vi "RT Loop - Acquisition and Logging.vi"(8 "error in (no error)":errorcluster, 9 "Acquisition and Logging Configuration":T1={"Data Rate"=1, "Samples per Read"=0, "Number of Reads to Save"=0, "Data File Name"="", "TDMS Properties"=[], "Number of Channels"=4, "Channel Scale Array"=[0.0, 0.0, 0.0, 0.0, 1.0, 1.0, 1.0, 1.0], "Channel Names"=[], "Trigger - RMS Value"=0.0, "Trigger - Channel"=0, "Trigger - Time (Minute)"=0} {"Data Rate" items=["51.200 kS/s (NI 9234)"=1, "25.600 kS/s (NI 9234)"=2, "17.067 kS/s (NI 9234)"=3, "12.800 kS/s (NI 9234)"=4, "10.240 kS/s (NI 9234)"=5, "8.533 kS/s (NI 9234)"=6, "7.314 kS/s (NI 9234)"=7, "6.400 kS/s (NI 9234)"=8, "5.689 kS/s (NI 9234)"=9, "5.120 kS/s (NI 9234)"=10, "4.654 kS/s (NI 9234)"=11, "4.267 kS/s (NI 9234)"=12, "3.938 kS/s (NI 9234)"=13, "3.657 kS/s (NI 9234)"=14, "3.413 kS/s (NI 9234)"=15, "3.200 kS/s (NI 9234)"=16, "3.012 kS/s (NI 9234)"=17, "2.845 kS/s (NI 9234)"=18, "2.695 kS/s (NI 9234)"=19, "2.560 kS/s (NI 9234)"=20, "2.438 kS/s (NI 9234)"=21, "2.328 kS/s (NI 9234)"=22, "2.226 kS/s (NI 9234)"=23, "2.133 kS/s (NI 9234)"=24, "2.048 kS/s (NI 9234)"=25, "1.969 kS/s (NI 9234)"=26, "1.896 kS/s (NI 9234)"=27, "1.829 kS/s (NI 9234)"=28, "1.765 kS/s (NI 9234)"=29, "1.707 kS/s (NI 9234)"=30, "1.652 kS/s (NI 9234)"=31]}, 10 "Acquisition and Logging Queue":refnum<queue>, 11 "Message Queue":refnum<queue>) -> ()   [LabVIEW 2015]
uses:
  controls/FPGA VI Reference.ctl
  support/Message Queue/Message Queue.lvlib
  Globals/Global - Configuration Options.vi
  Globals/Global - Monitoring Variables.vi
  support/Message Queue/Message Cluster.ctl
  controls/Acquisition and Logging Configuration.ctl
  <vilib>/LabVIEW Targets/FPGA/cRIO/shared/nicrio_ModuleControls/nicrio_cRIO-9234_DataRatesRing2.ctl
  controls/TDMS Properties.ctl
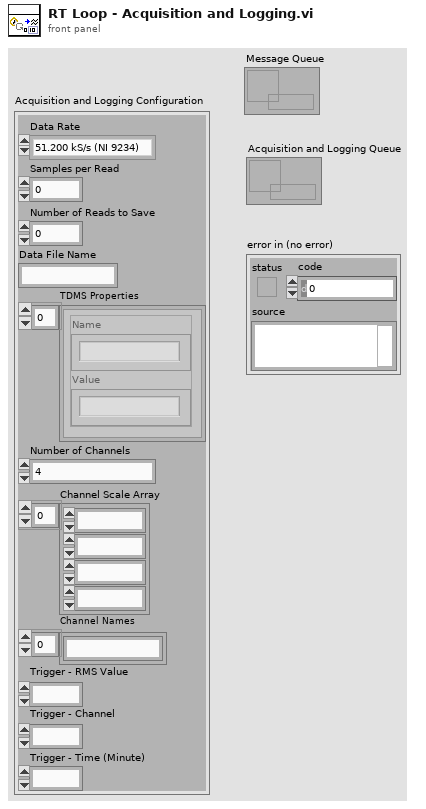
[diagram p1: front panel]
types:
  T1 = typedef "Acquisition and Logging Configuration.ctl" = cluster{"Data Rate":T2, "Samples per Read":i32, "Number of Reads to Save":i32, "Data File Name":string, "TDMS Properties":T3[], "Number of Channels":i32, "Channel Scale Array":fxp<+,24,12>[], "Channel Names":string[], "Trigger - RMS Value":dbl, "Trigger - Channel":i32, "Trigger - Time (Minute)":i32}
  T2 = typedef "nicrio_cRIO-9234_DataRatesRing2.ctl" = u8
  T3 = typedef "TDMS Properties.ctl" = cluster{"Name":string, "Value":string}
  T4 = typedef "FPGA VI Reference.ctl" = refnum<k20>
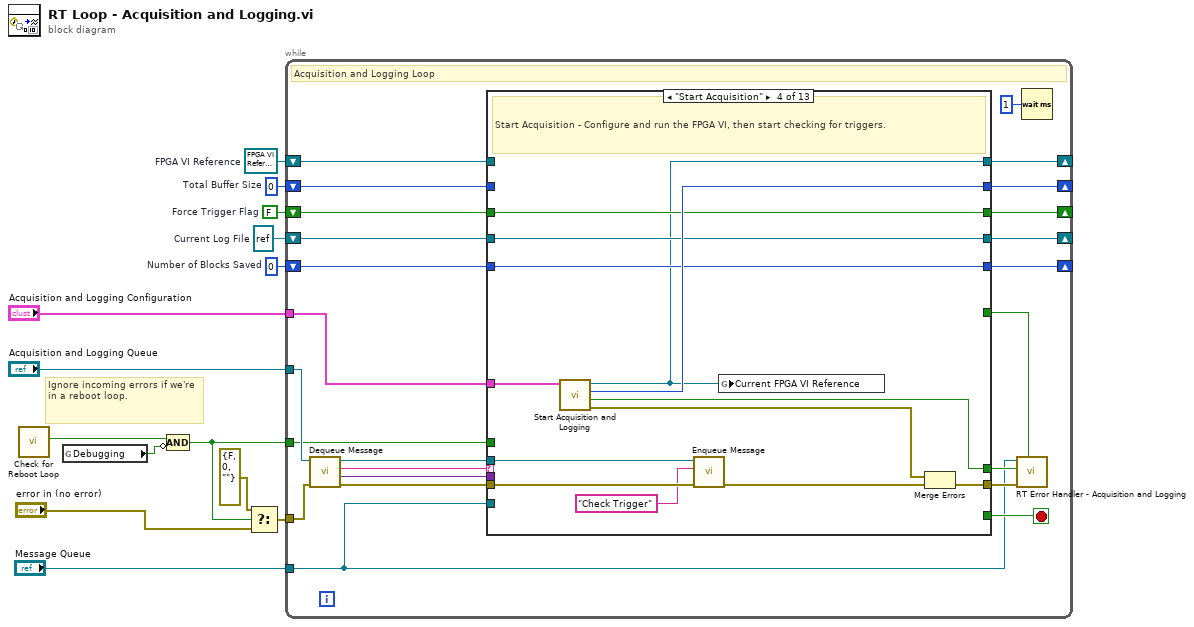
[diagram p0: block diagram]
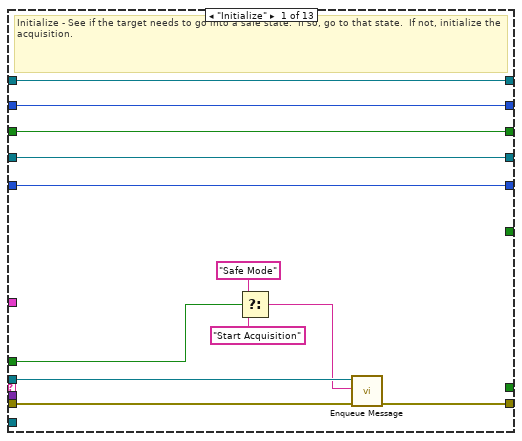
[diagram p2: hidden frame]
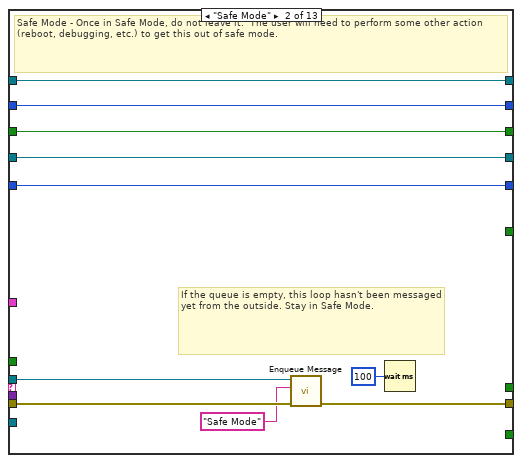
[diagram p3: hidden frame]
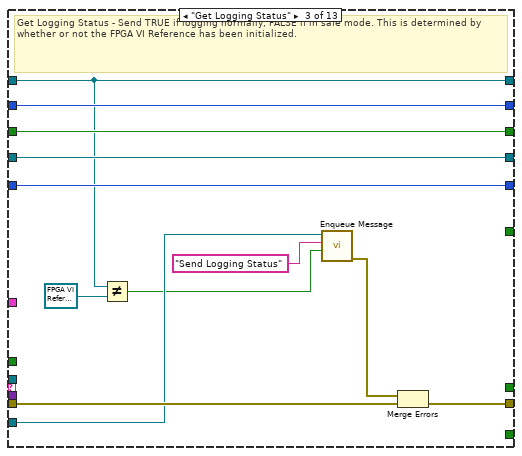
[diagram p4: hidden frame]
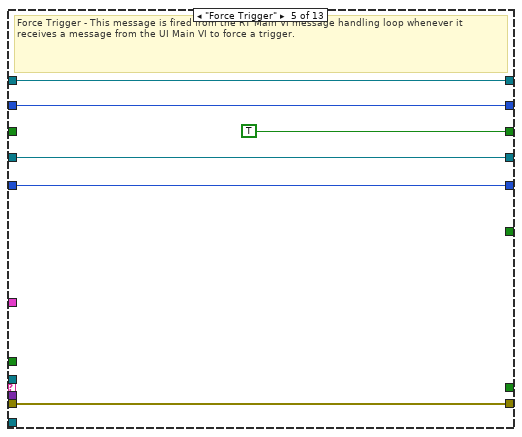
[diagram p5: hidden frame]
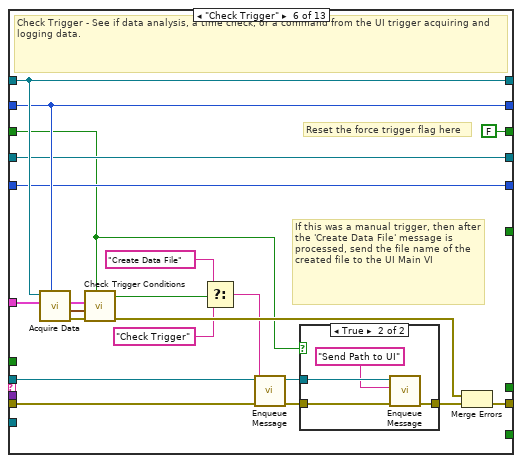
[diagram p6: hidden frame]
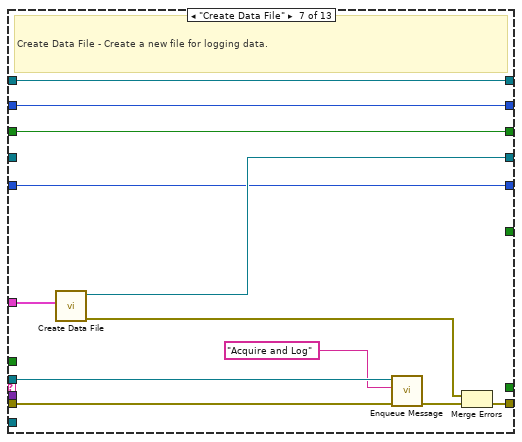
[diagram p8: hidden frame]
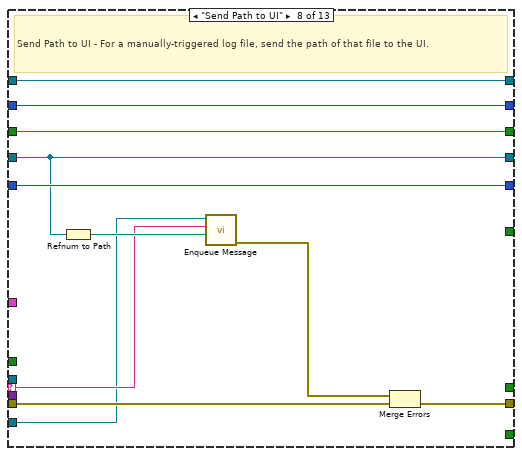
[diagram p9: hidden frame]
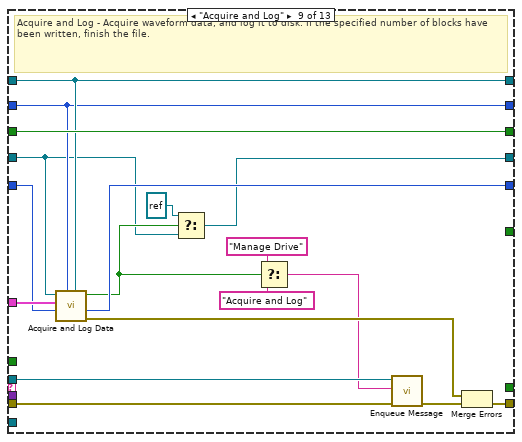
[diagram p10: hidden frame]
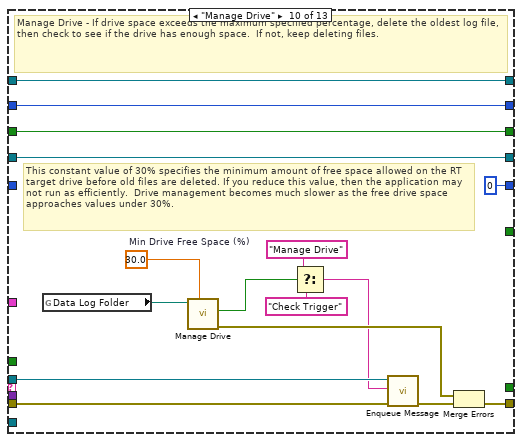
[diagram p11: hidden frame]
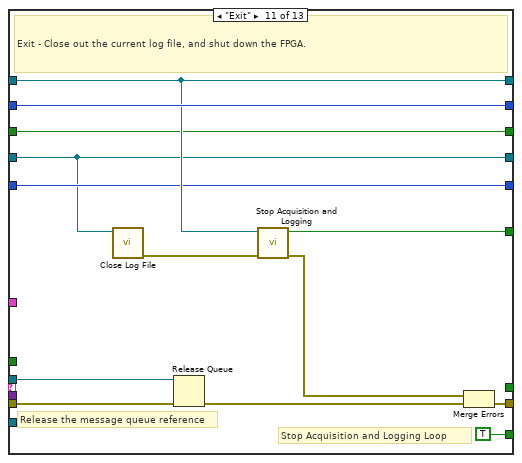
[diagram p12: hidden frame]
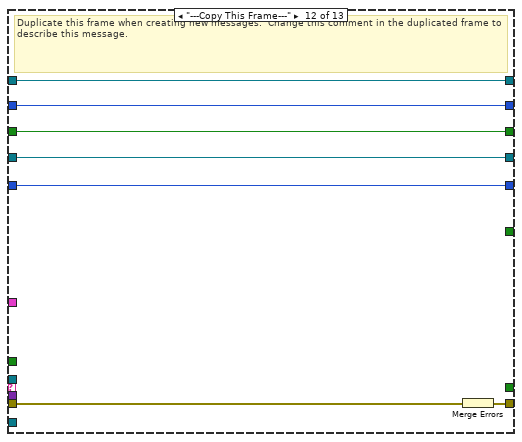
[diagram p13: hidden frame]
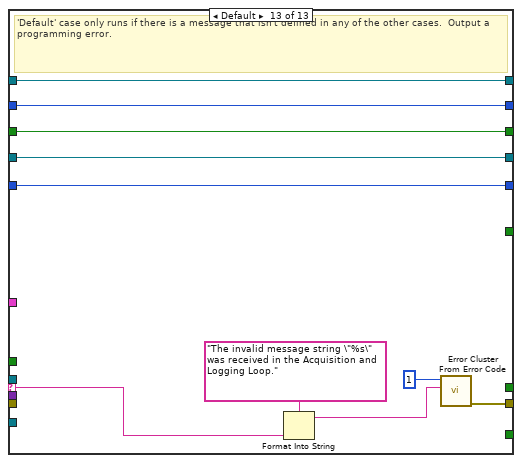
[diagram p14: hidden frame]
diagram:
  w7 = 0  # Number of Blocks Saved
  w8 = refnum<k34> refnum  # Current Log File
  w9 = FALSE  # Force Trigger Flag
  w11 = 0  # Total Buffer Size
  w12 = T4 refnum  # FPGA VI Reference
  # "Ignore incoming errors if we're in a reboot loop."
  n1 = call "Check for Reboot Loop.vi"() -> ("Start in Safe Mode?"=w3:bool)  [unwired: 10 in, 1 out]
  n2 = global read "Global - Configuration Options.vi" "Debugging"() -> (w2:bool)
  n3 = Compound Arithmetic op=AND(w3, invert w2) -> (w1:bool)
  n4 = Select(t=errorcluster {"status"=FALSE, "code"=0, "source"=""}, s=w1, f="error in (no error)") -> (s? t:f=w5:errorcluster)
  n5 = while {
    tunnel: "Acquisition and Logging Queue" -> [w34]
    tunnel: "Message Queue" -> [w18]
    shift-right: [w29] -> _
    shift-left: w12 -> [w31]
    shift-right: [w28] -> _
    shift-left: w11 -> [w30]
    tunnel: "Acquisition and Logging Configuration" -> [w27]
    shift-right: [w23] -> _
    shift-left: w9 -> [w24]
    shift-right: [w21] -> _
    shift-left: w8 -> [w22]
    shift-right: [w19] -> _
    shift-left: w7 -> [w20]
    tunnel: w5 -> [w16]
    tunnel: w1 -> [w15]
    stop <- w38 stop-if-true
    # "Acquisition and Logging Loop"
    n6 = call "Dequeue Message.vi"("error in (no error)"=w16, "Message Queue"=w34) -> ("error out"=w37:errorcluster, "Message Data"=w35:variant, "Message"=w36:string, "dup Message Queue"=w32:refnum<queue>)  [unwired: 6 in]
    n7 = case "Message Cases" shown="\"Start Acquisition\"" w36 {
      selector: w36 -> [_ _ _ _ _ _ _ w133 _ _ _ _ w203]
      tunnel: w32 -> [w47 w57 _ w78 _ w103 w124 _ w155 w167 w187 _ _]
      tunnel: w37 -> [w48 w58 w72 w85 w91 w111 w128 w140 w158 w174 w183 w194 _]
      tunnel: [w40 w56 w64 w83 w91 w110 w127 w131 w157 w170 w184 w193 w201] -> w33
      tunnel: [_ _ _ _ _ _ _ _ _ _ TRUE _ _] -> w38
      tunnel: w35 -> [_ _ _ _ _ _ _ _ _ _ _ _ _]
      tunnel: w31 -> [w50 w60 w67 _ w90 w112 w129 w139 w148 w173 w181 w192 w199]
      tunnel: w30 -> [w49 w59 w71 _ w89 w108 w126 w138 w147 w172 w182 w191 w198]
      tunnel: [w50 w60 w67 w73 w90 w112 w129 w139 w148 w173 w181 w192 w199] -> w29
      tunnel: [w49 w59 w71 w80 w89 w108 w126 w138 w147 w172 w182 w191 w198] -> w28
      tunnel: w27 -> [_ _ _ w84 _ w109 w121 _ w153 _ _ _ _]
      tunnel: [_ _ _ w81 _ _ _ _ _ _ _ _ _] -> w25
      tunnel: w24 -> [w43 w55 w70 w76 _ w92 w122 w137 w154 w160 w179 w190 w197]
      tunnel: [w43 w55 w70 w76 TRUE ("Force Trigger Flag") FALSE ("Force Trigger Flag") w122 w137 w154 w160 w179 w190 w197] -> w23
      tunnel: w22 -> [w42 w54 w69 w75 w88 w98 _ w135 w143 w171 w176 w189 w196]
      tunnel: [w42 w54 w69 w75 w88 w98 w119 w135 w142 w171 w176 w189 w196] -> w21
      tunnel: w20 -> [w41 w53 w68 w74 w86 w97 w118 w136 w146 _ w178 w188 w195]
      tunnel: [w41 w53 w68 w74 w86 w97 w118 w136 w145 0 ("Number of Blocks Saved") w178 w188 w195] -> w19
      tunnel: w18 -> [_ _ w65 _ _ _ _ w132 _ _ _ _ _]
      tunnel: [_ _ _ _ _ _ _ _ _ _ w175 _ _] -> w17
      tunnel: w15 -> [w39 _ _ _ _ _ _ _ _ _ _ _ _]
      frame "Initialize" {
        # "Initialize - See if the target needs to go into a safe state.  If so, go to that state.  If not, initialize the acquisition."
        n8 = Select(t="Safe Mode", s=w39, f="Start Acquisition") -> (s? t:f=w44:string)
        n9 = call "Enqueue Message.vi"("error in (no error)"=w48, "Message"=w44, "Message Queue"=w47) -> ("error out"=w40:errorcluster)  [unwired: 7 in, 1 out]
      }
      frame "Safe Mode" {
        # "If the queue is empty, this loop hasn't been messaged yet from the outside. Stay in Safe Mode."
        # "Safe Mode - Once in Safe Mode, do not leave it.  The user will need to perform some other action (reboot, debugging, etc.) to get this out of safe mode."
        n10 = call "Enqueue Message.vi"("error in (no error)"=w58, "Message"="Safe Mode", "Message Queue"=w57) -> ("error out"=w56:errorcluster)  [unwired: 7 in, 1 out]
        n11 = Wait (ms)(milliseconds to wait=u32 100) -> ()  [unwired: 1 out]
      }
      frame "Get Logging Status" {
        # "Get Logging Status - Send TRUE if logging normally, FALSE if in safe mode. This is determined by whether or not the FPGA VI Reference has been initialized."
        n12 = Not Equal?(x=w67, y=T4 refnum ("FPGA VI Reference")) -> (x != y?=w62:bool)
        n13 = call "Enqueue Message.vi"("Message Data"=w62, "Message"="Send Logging Status", "Message Queue"=w65) -> ("error out"=w63:errorcluster)  [unwired: 7 in, 1 out]
        n14 = Merge Errors(w63, w72) -> (w64:errorcluster)
      }
      frame "Start Acquisition" {
        # "Start Acquisition - Configure and run the FPGA VI, then start checking for triggers."
        n15 = call "Start Acquisition and Logging.vi"("Acquisition and Logging Configuration"=w84) -> ("error out"=w82:errorcluster, "Wait on IRQ Timeout?"=w81:bool, "Total Buffer Size"=w80:i32, "FPGA VI Reference Out"=w73:T4)  [unwired: 7 in]
        n16 = call "Enqueue Message.vi"("error in (no error)"=w85, "Message"="Check Trigger", "Message Queue"=w78) -> ("error out"=w79:errorcluster)  [unwired: 7 in, 1 out]
        n17 = global write "Global - Monitoring Variables.vi" "Current FPGA VI Reference"(w73) -> ()
        n18 = Merge Errors(w82, w79) -> (w83:errorcluster)
      }
      frame "Force Trigger" {
        # "Force Trigger - This message is fired from the RT Main VI message handling loop whenever it receives a message from the UI Main VI to force a trigger."
      }
      frame "Check Trigger" {
        # "If this was a manual trigger, then after the 'Create Data File' message is processed, send the file name of the created file to the UI Main VI"
        # "Reset the force trigger flag here"
        # "Check Trigger - See if data analysis, a time check, or a command from the UI trigger acquiring and logging data."
        n19 = call "Acquire Data.vi"("Total Buffer Size"=w108, "Acquisition and Logging Configuration"=w109, "FPGA VI Reference"=w112) -> ("error out"=w106:errorcluster, "Waveform Data"=w105:waveform(sgl)[], "dup Acquisition and Logging Configuration"=w104:T1)  [unwired: 6 in]
        n20 = call "Check Trigger Conditions.vi"("Force Trigger?"=w92, "error in (no error)"=w106, "Waveform Data"=w105, "Acquisition and Logging Configuration"=w104) -> ("error out"=w107:errorcluster, "Trigger Condition Met?"=w102:bool)  [unwired: 6 in]
        n21 = Select(t="Create Data File", s=w102, f="Check Trigger") -> (s? t:f=w99:string)
        n22 = call "Enqueue Message.vi"("error in (no error)"=w111, "Message"=w99, "Message Queue"=w103) -> ("error out"=w95:errorcluster, "dup Message Queue"=w93:refnum<queue>)  [unwired: 7 in]
        n23 = case shown="True" w92 {
          tunnel: w95 -> [w113 w116]
          tunnel: [w113 w117] -> w94
          tunnel: w93 -> [_ w115]
          frame False {
          }
          frame True {
            n24 = call "Enqueue Message.vi"("error in (no error)"=w116, "Message"="Send Path to UI", "Message Queue"=w115) -> ("error out"=w117:errorcluster)  [unwired: 7 in, 1 out]
          }
        }
        n25 = Merge Errors(w107, w94) -> (w110:errorcluster)
      }
      frame "Create Data File" {
        # "Create Data File - Create a new file for logging data."
        n26 = call "Create Data File.vi"("Acquisition and Logging Configuration"=w121) -> ("error out"=w120:errorcluster, "TDMS File Reference"=w119:refnum<k34>)  [unwired: 9 in]
        n27 = call "Enqueue Message.vi"("error in (no error)"=w128, "Message"="Acquire and Log", "Message Queue"=w124) -> ("error out"=w125:errorcluster)  [unwired: 7 in, 1 out]
        n28 = Merge Errors(w120, w125) -> (w127:errorcluster)
      }
      frame "Send Path to UI" {
        # "Send Path to UI - For a manually-triggered log file, send the path of that file to the UI."
        n29 = Refnum to Path(1:w135) -> (0:w134:path)
        n30 = call "Enqueue Message.vi"("Message Data"=w134, "Message"=w133, "Message Queue"=w132) -> ("error out"=w130:errorcluster)  [unwired: 7 in, 1 out]
        n31 = Merge Errors(w130, w140) -> (w131:errorcluster)
      }
      frame "Acquire and Log" {
        # "Acquire and Log - Acquire waveform data, and log it to disk. If the specified number of blocks have been written, finish the file."
        n32 = call "Acquire and Log Data.vi"("FPGA VI Reference"=w148, "Total Buffer Size"=w147, "Number of Blocks Saved in"=w146, "Acquisition and Logging Configuration"=w153, "TDMS File Reference"=w143) -> ("error out"=w152:errorcluster, "Number of Blocks Saved out"=w145:i32, "Logging Complete?"=w144:bool)  [unwired: 4 in]
        n33 = Select(t=refnum<k34> refnum, s=w144, f=w143) -> (s? t:f=w142:refnum<k34>)
        n34 = Select(t="Manage Drive", s=w144, f="Acquire and Log") -> (s? t:f=w149:string)
        n35 = call "Enqueue Message.vi"("error in (no error)"=w158, "Message"=w149, "Message Queue"=w155) -> ("error out"=w156:errorcluster)  [unwired: 7 in, 1 out]
        n36 = Merge Errors(w152, w156) -> (w157:errorcluster)
      }
      frame "Manage Drive" {
        w169 = 30.0  # Min Drive Free Space (%)
        # "This constant value of 30% specifies the minimum amount of free space allowed on the RT target drive before old files are deleted. If you reduce this value, then the application may not run as efficiently.  Drive management becomes much slower as the free drive space approaches values under 30%."
        # "Manage Drive - If drive space exceeds the maximum specified percentage, delete the oldest log file, then check to see if the drive has enough space.  If not, keep deleting files."
        n37 = global read "Global - Configuration Options.vi" "Data Log Folder"() -> (w159:path)
        n38 = call "Manage Drive.vi"("Min Drive Free Space (%)"=w169, "Data Folder"=w159) -> ("error out"=w166:errorcluster, "Drive Space Below Limit"=w165:bool)  [unwired: 8 in]
        n39 = Select(t="Manage Drive", s=w165, f="Check Trigger") -> (s? t:f=w162:string)
        n40 = call "Enqueue Message.vi"("error in (no error)"=w174, "Message"=w162, "Message Queue"=w167) -> ("error out"=w168:errorcluster)  [unwired: 7 in, 1 out]
        n41 = Merge Errors(w166, w168) -> (w170:errorcluster)
      }
      frame "Exit" {
        # "Stop Acquisition and Logging Loop"
        # "Release the message queue reference"
        # "Exit - Close out the current log file, and shut down the FPGA."
        n42 = call "Close Log File.vi"("Log File"=w176) -> ("error out"=w177:errorcluster)  [unwired: 10 in]
        n43 = Release Queue(queue=w187, error in (no error)=w183) -> (error out=w185:errorcluster)  [unwired: 1 in, 2 out]
        n44 = call "Stop Acquisition and Logging.vi"("error in (no error)"=w177, "FPGA VI Reference"=w181) -> ("error out"=w180:errorcluster, "Stop FPGA Timeout?"=w175:bool)  [unwired: 8 in]
        n45 = Merge Errors(w180, w185) -> (w184:errorcluster)
      }
      frame "---Copy This Frame---" {
        # "Duplicate this frame when creating new messages.  Change this comment in the duplicated frame to describe this message."
        n46 = Merge Errors(w194) -> (w193:errorcluster)
      }
      frame Default {
        # "'Default' case only runs if there is a message that isn't defined in any of the other cases.  Output a programming error."
        n47 = Format Into String(format string="The invalid message string \"%s\" was received in the Acquisition and Logging Loop." ("Unknown Message Error Text"), w203) -> (resulting string=w200:string)  [unwired: 2 in, 1 out]
        n48 = call <vilib>:"Error Cluster From Error Code.vi"("error message (\"\")"=w200, "error code (0)"=1) -> ("error out"=w201:errorcluster)  [unwired: 7 in]
      }
    }
    n49 = call "RT Error Handler - Acquisition and Logging.vi"("Stop FPGA Timeout"=w17, "error in (no error)"=w33, "IRQ Timeout"=w25, "Message Queue"=w18) -> ()  [unwired: 7 in, 1 out]
    n50 = Wait (ms)(milliseconds to wait=u32 1) -> ()  [unwired: 1 out]
  }
